vi "F Dwf Analog In Status Noise.vi"(6 "cdData":i32, 7 "rgdMax":dbl, 8 "error in (no error)":errorcluster, 9 "rgdMin":dbl, 10 "idxChannel":i32, 11 "hdwf":i32) -> (0 "error out":errorcluster, 1 "rgdMin out":dbl, 3 "function return":i32, 5 "rgdMax out":dbl)   [LabVIEW 2021, in "Olasdwf.lvlib"]
doc: "DWFAPI int FDwfAnalogInStatusNoise(HDWF hdwf, int idxChannel, double *rgdMin, double *rgdMax, int cdData);"
uses:
  Olasdwf.lvlib
  Windows/System32/dwf.dll
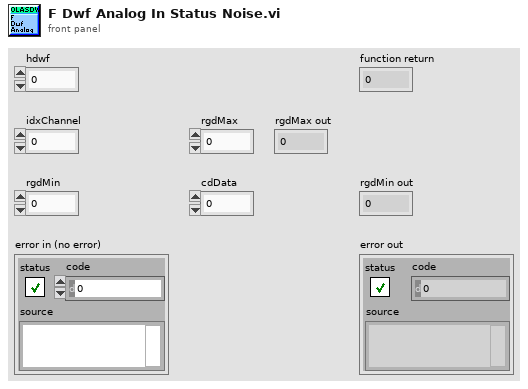
[diagram p1: front panel]
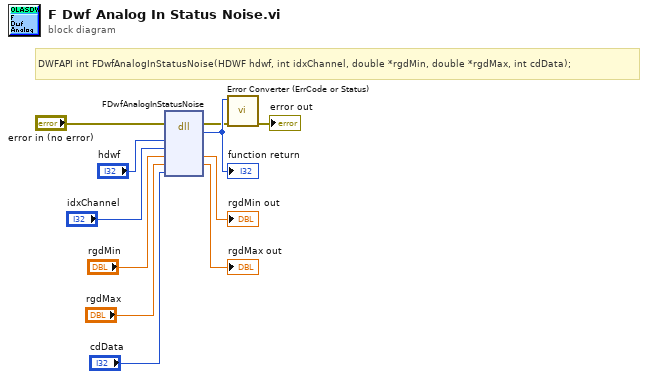
[diagram p0: block diagram]
diagram:
  # "DWFAPI int FDwfAnalogInStatusNoise(HDWF hdwf, int idxChannel, double *rgdMin, double *rgdMax, int cdData);"
  n1 = dll-call lib="/Windows/System32/dwf.*" fn="FDwfAnalogInStatusNoise"(error in="error in (no error)", "hdwf"="hdwf", "idxChannel"="idxChannel", "rgdMin"="rgdMin", "rgdMax"="rgdMax", "cdData"="cdData") -> (error out=w2:errorcluster, w11:i32, "rgdMin"=→"rgdMin out":dbl, "rgdMax"=→"rgdMax out":dbl)  [unwired: 5 in, 1 out]
  "function return" <- w11
  n2 = call "Error Converter (ErrCode or Status).vi"("error in (no error)"=w2, "error code"=w11) -> ("error out"=→"error out":errorcluster)  [unwired: 9 in]
